vi "NanotecSMCPDDriver.set positioning mode.vi"(0 "VISA resource name":refnum<visa-resource-name>, 1 "contollerID":i32=-1, 3 "positioningMode":T1, 5 "error in (no error)":errorcluster) -> (14 "VISA resource name out":refnum<visa-resource-name>, 15 "contollerID out":i32=-1, 19 "error out":errorcluster)   [LabVIEW 2014, in "NanotecSMCPDDriver.lvlib"]
doc: "Sets the positioning mode of the controller (absolute, relative, ...)"
uses:
  NanotecSMCPDDriver.lvlib
  NanotecSMCPDDriver.positioning mode types.ctl
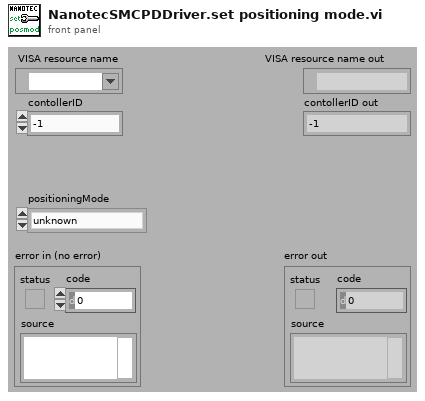
[diagram p1: front panel]
types:
  T1 = typedef "NanotecSMCPDDriver.lvlib/NanotecSMCPDDriver.positioning mode types.ctl" = enum16{"unknown", "relative positioning", "absolute positioning", "internal referencing", "external referencing"}
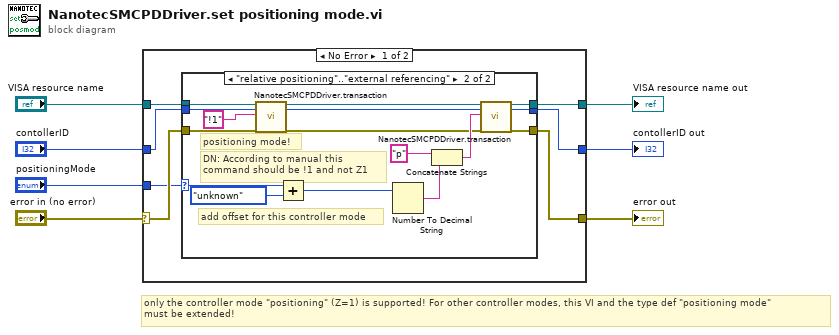
[diagram p0: block diagram]
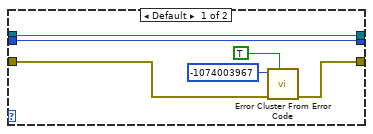
[diagram p2: hidden frame]
diagram:
  # "only the controller mode \"positioning\" (Z=1) is supported! For other controller modes, this VI and the type def \"positioning mode\"\nmust be extended!"
  n1 = case shown="No Error" "error in (no error)" {
    selector: "error in (no error)" -> [w9 w37]
    tunnel: [w13 w39] -> w7
    tunnel: [w12 w37] -> w6
    tunnel: "VISA resource name" -> [w11 w39]
    tunnel: "contollerID" -> [w10 w38]
    tunnel: [w14 w38] -> w3
    tunnel: "positioningMode" -> [w8 _]
    frame No Error {
      n2 = case shown="\"relative positioning\"..\"external referencing\"" w8 {
        selector: w8 -> [_ w30]
        tunnel: w11 -> [w20 w29]
        tunnel: w10 -> [w15 w27]
        tunnel: [w15 w36] -> w14
        tunnel: [w20 w35] -> w13
        tunnel: [w19 w34] -> w12
        tunnel: w9 -> [w18 w28]
        frame Default {
          n3 = call <vilib>:"Error Cluster From Error Code.vi"("show call chain? (False)"=TRUE, "error in (no error)"=w18, "error code (0)"=-1074003967) -> ("error out"=w19:errorcluster)  [unwired: 6 in]
        }
        frame "relative positioning".."external referencing" {
          # "DN: According to manual this \ncommand should be !1 and not Z1"
          # "add offset for this controller mode"
          # "positioning mode!"
          n4 = call "NanotecSMCPDDriver.transaction.vi"("VISAresource"=w29, "contollerID"=w27, "commandString"="!1", "error in (no error)"=w28) -> ("VISAresource out"=w23:refnum<visa-resource-name>, "contollerID out"=w22:i32, "error out"=w21:errorcluster)  [unwired: 10 in, 3 out]
          n5 = Add(x=w30, y=NanotecSMCPDDriver.positioning_mode_types."unknown") -> (x+y=w24:u16)
          n6 = Number To Decimal String(number=w24) -> (decimal integer string=w33:string)  [unwired: 1 in]
          n7 = Concatenate Strings("p" ("commandString"), w33) -> (w31:string)
          n8 = call "NanotecSMCPDDriver.transaction.vi"("VISAresource"=w23, "contollerID"=w22, "commandString"=w31, "error in (no error)"=w21) -> ("VISAresource out"=w35:refnum<visa-resource-name>, "contollerID out"=w36:i32, "error out"=w34:errorcluster)  [unwired: 10 in, 3 out]
        }
      }
    }
    frame Error {
    }
  }
  "VISA resource name out" <- w7
  "error out" <- w6
  "contollerID out" <- w3
